vi "volume integrator.vi"(4 "Previous Time (msec)":u32, 6 "Flow":dbl format="%.2f", 7 "Total Volume in":dbl format="%.2f") -> (0 "Current Time (msec)":u32, 3 "Total Volume Out":dbl format="%.2f")   [LabVIEW 2016]
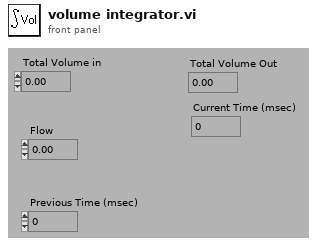
[diagram p1: front panel]
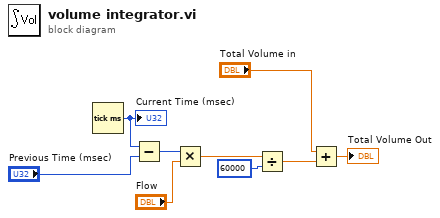
[diagram p0: block diagram]
diagram:
  n1 = Tick Count (ms)() -> (millisecond timer value=w7:u32)
  "Current Time (msec)" <- w7
  n2 = Subtract(x=w7, y="Previous Time (msec)") -> (x-y=w8:u32)
  n3 = Multiply(x=w8, y="Flow") -> (x*y=w1:dbl)
  n4 = Divide(x=w1, y=60000) -> (x/y=w2:dbl)
  n5 = Add(x="Total Volume in", y=w2) -> (x+y=→"Total Volume Out":dbl)
